vi "SendTCP-IP.vi"(8 "error in (no error)":errorcluster, 9 "Data":variant, 10 "connection in":T1, 11 "Control in":refnum<class "Control-Server.lvclass">) -> (0 "error out":errorcluster, 3 "Control out":refnum<class "Control-Server.lvclass">)   [LabVIEW 2015, in "Control-Server.lvclass"]
uses:
  Control-Server.lvclass
  <vilib>/NI/STM/TCP/TCP Connection Info.ctl
  <vilib>/NI/STM/SubVIs/MetaDataElement.ctl
  dependecies/ControlsVIs/Clusters-def/Standard Command.ctl
  <vilib>/NI/STM/Connection Manager/TCP/TCP Connection Method.ctl
  <vilib>/NI/STM/TCP/Write Message (TCP).vi
  <vilib>/NI/STM/NI STM.lvlib
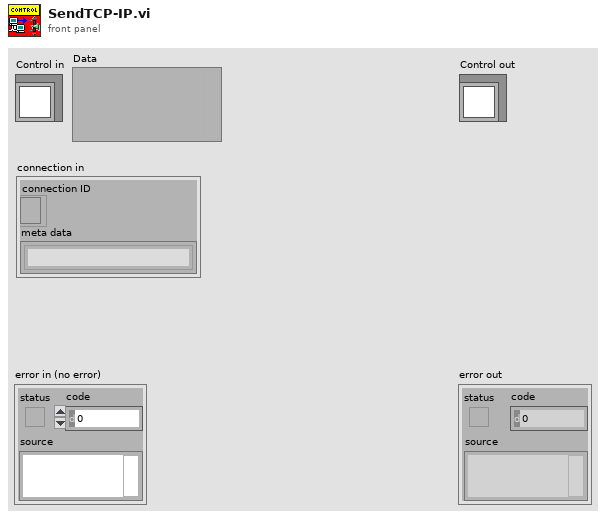
[diagram p1: front panel]
types:
  T1 = typedef "NI STM.lvlib/TCP Connection Info.ctl" = cluster{"connection ID":refnum<k5>, "meta data":T2[]}
  T2 = typedef "NI STM.lvlib/MetaDataElement.ctl" = string
  T3 = typedef "NI STM.lvlib/TCP Connection Method.ctl" = enum16{"Initialize", "Add Connection", "Set Properties", "Get Connection(s)", "Remove Connection", "Remove All Connections", "Get Connection Count"}
  T4 = typedef "Standard Command.ctl" = cluster{"command":string, "data":variant}
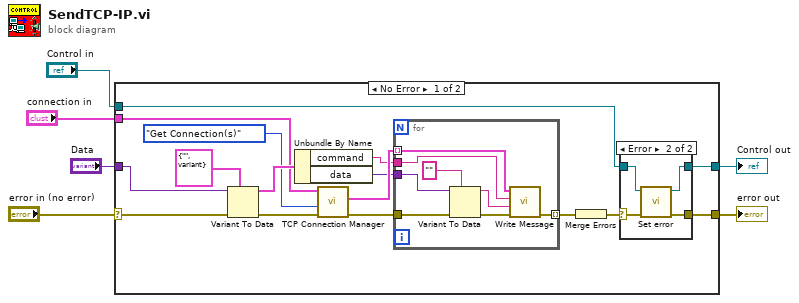
[diagram p0: block diagram]
diagram:
  n1 = case shown="No Error" "error in (no error)" {
    selector: "error in (no error)" -> [w9 w37]
    tunnel: "Data" -> [w20 _]
    tunnel: "connection in" -> [w19 _]
    tunnel: [w12 w37] -> w6
    tunnel: "Control in" -> [w7 w38]
    tunnel: [w10 w38] -> w1
    frame No Error {
      n2 = Variant To Data(error in=w9, type=T4 {"command"="", "data"=variant} ("input cluster"), Variant=w20) -> (data=w22:T4, error out=w8:errorcluster)
      n3 = Unbundle By Name(w22) -> ("command"=w13:string, "data"=w14:variant)
      n4 = call <vilib>:"TCP Connection Manager.vi"("error in"=w8, "method"=TCP_Connection_Method."Get Connection(s)", "connection in"=w19) -> ("error out"=w16:errorcluster, "all connections"=w18:T1[])  [unwired: 3 in, 4 out]
      n5 = for {
        tunnel: [w29] -> w15 mode=indexing
        tunnel: w18 -> [w35] mode=indexing
        tunnel: w16 -> [w36]
        tunnel: w14 -> [w31]
        tunnel: w13 -> [w34]
        n6 = Variant To Data(error in=w36, type="" ("*(type *) &x"), Variant=w31) -> (data=w32:string, error out=w30:errorcluster)
        n7 = call-poly <vilib>:"Write Message.vi"("error in"=w30, "data"=w32, "name"=w34, "connection info in"=w35) -> ("error out"=w29:errorcluster)  [unwired: 6 in, 1 out]
      }
      n8 = Merge Errors(w15) -> (w11:errorcluster)
      n9 = case shown="Error" w11 {
        selector: w11 -> [w24 w26]
        tunnel: w7 -> [w23 w28]
        tunnel: [w24 w27] -> w12
        tunnel: [w23 w25] -> w10
        frame No Error {
        }
        frame Error {
          n10 = call "Set error.vi"("error in (no error)"=w26, "Control-Server in"=w28) -> ("error out"=w27:errorcluster, "Control-Server out"=w25:refnum<class "Control-Server.lvclass">)  [unwired: 8 in]
        }
      }
    }
    frame Error {
    }
  }
  "error out" <- w6
  "Control out" <- w1
